vi "Autonomous Commands Latches and Toggles.vi"(1 "Robot System Functions":T1) -> (0 "Robot System Functions Output":T1)   [LabVIEW 2014]
uses:
  Subsystems VIs/Robot Commands.ctl
panel:
  # "The Purpose of this VI is to simulate how the Input to Commands.vi in Teleop Functions"
  # "Field Centric"
  # "Field Centric"
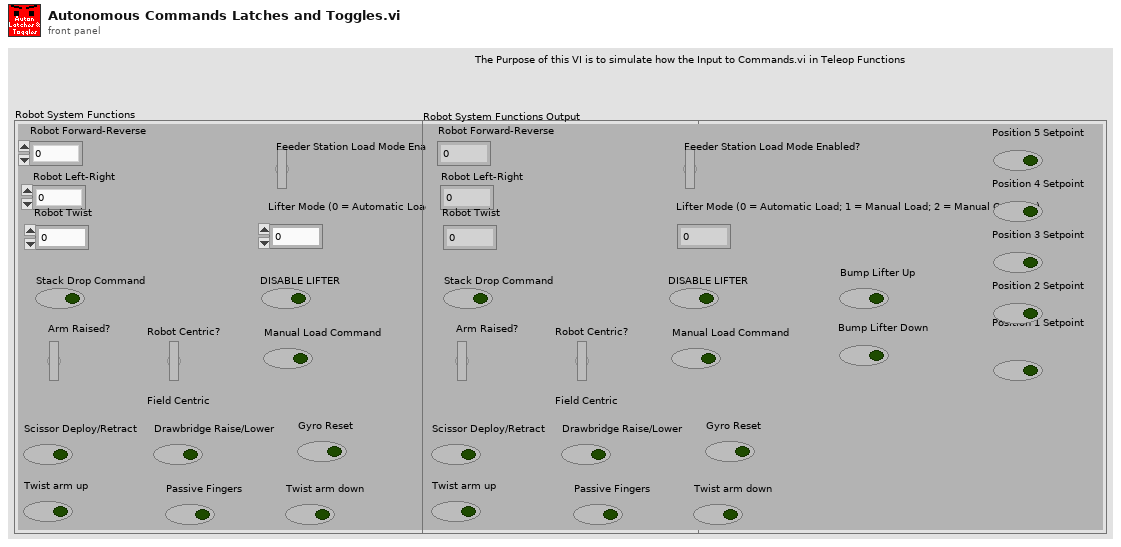
[diagram p1: front panel]
types:
  T1 = typedef "Robot Commands.ctl" = cluster{"Robot Forward-Reverse":dbl, "Robot Left-Right":dbl, "Robot Twist":dbl, "Feeder Station Load Mode Enabled?":bool, "Lifter Mode (0 = Automatic Load; 1 = Manual Load; 2 = Manual Override)":dbl, "Stack Drop Command":bool, "Arm Raised?":bool, "DISABLE LIFTER":bool, "Position 1 Setpoint":bool, "Position 2 Setpoint":bool, "Position 3 Setpoint":bool, "Position 4 Setpoint":bool, "Position 5 Setpoint":bool, "Bump Lifter Down":bool, "Bump Lifter Up":bool, "Manual Load Command":bool, "Robot Centric?":bool, "Scissor Deploy/Retract":bool, "Passive Fingers":bool, "Drawbridge Raise/Lower":bool, "Twist arm up":bool, "Gyro Reset":bool, "Twist arm down":bool}
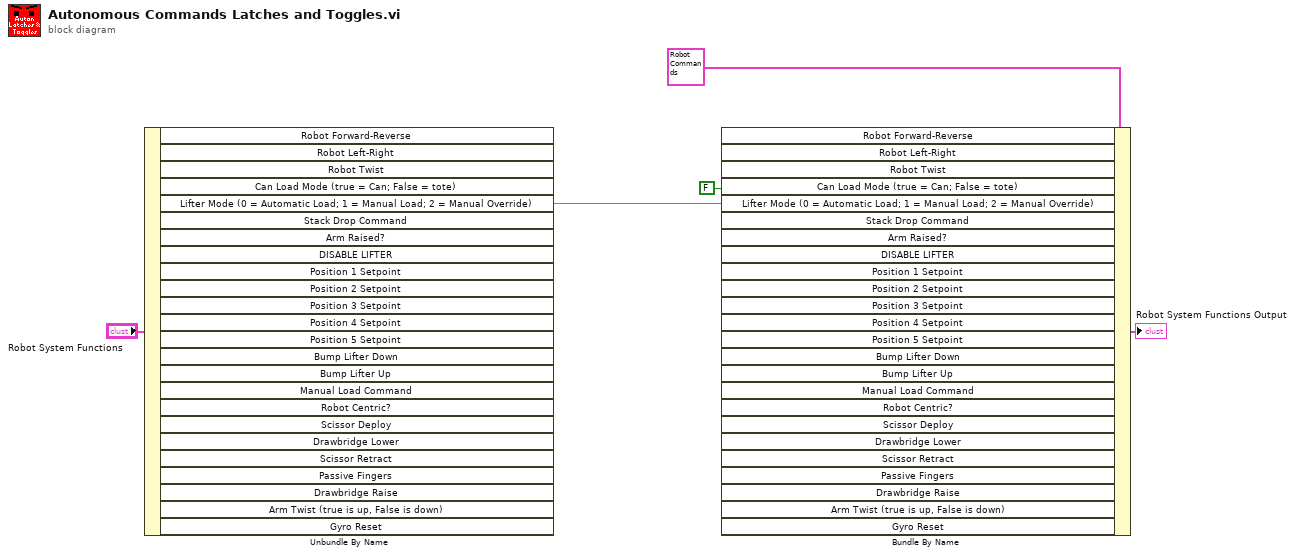
[diagram p0: block diagram]
diagram:
  n1 = Unbundle By Name("Robot System Functions") -> ("Lifter Mode (0 = Automatic Load; 1 = Manual Load; 2 = Manual Override)"=w1:dbl)  [unwired: 23 out]
  n2 = Bundle By Name(cluster=T1 {"Robot Forward-Reverse"=0.0, "Robot Left-Right"=0.0, "Robot Twist"=0.0, "Feeder Station Load Mode Enabled?"=FALSE, "Lifter Mode (0 = Automatic Load; 1 = Manual Load; 2 = Manual Override)"=0.0, "Stack Drop Command"=FALSE, "Arm Raised?"=FALSE, "DISABLE LIFTER"=FALSE, "Position 1 Setpoint"=FALSE, "Position 2 Setpoint"=FALSE, "Position 3 Setpoint"=FALSE, "Position 4 Setpoint"=FALSE, "Position 5 Setpoint"=FALSE, "Bump Lifter Down"=FALSE, "Bump Lifter Up"=FALSE, "Manual Load Command"=FALSE, "Robot Centric?"=FALSE, "Scissor Deploy/Retract"=FALSE, "Passive Fingers"=FALSE, "Drawbridge Raise/Lower"=FALSE, "Twist arm up"=FALSE, "Gyro Reset"=FALSE, "Twist arm down"=FALSE} ("Robot System Functions 2"), "Can Load Mode (true = Can; False = tote)"=FALSE, "Lifter Mode (0 = Automatic Load; 1 = Manual Load; 2 = Manual Override)"=w1) -> (→"Robot System Functions Output":T1)  [unwired: 22 in]
